vi "Write S6F1.vi"(8 "error in (no error)":errorcluster, 10 "S6F1":T1, 11 "33-Update Trace Data in":refnum<class "33-Update Trace Data.lvclass">) -> (0 "error out":errorcluster, 3 "33-Update Trace Data out":refnum<class "33-Update Trace Data.lvclass">)   [LabVIEW 2020, in "SECS Scenarios.lvlib" / "33-Update Trace Data.lvclass"]
uses:
  33-Update Trace Data.lvclass
  SECS Communication/S6 Message Class/S6F1.ctl
  SECS Communication/SECS-II Class/Format Code.ctl
  33-Update Trace Data.lvclass/33-Update Trace Data.ctl
  SECS Communication/SECS-II Class/SECS-II Class.lvclass
  SECS Communication/S6 Message Class/S6 Message Class.lvclass
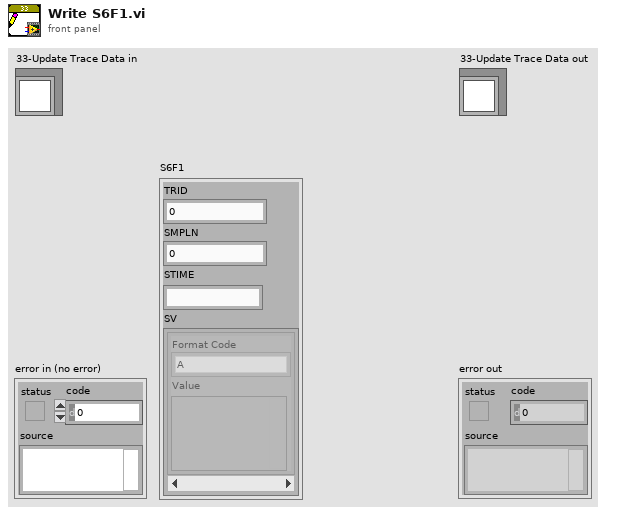
[diagram p1: front panel]
types:
  T1 = typedef "SECS Communication.lvlib/S6 Message Class.lvclass/S6F1.ctl" = cluster{"TRID":u32, "SMPLN":u32, "STIME":string, "SV":cluster{"Format Code":T2, "Value":variant}[]}
  T2 = typedef "SECS Communication.lvlib/SECS-II Class.lvclass/Format Code.ctl" = enum16{"L", "A", "B", "Boolean", "J", "I1", "I2", "I4", "I8", "U1", "U2", "U4", "U8", "F4", "F8", "Char"}
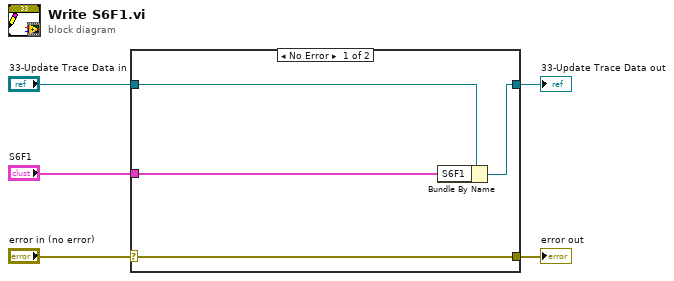
[diagram p0: block diagram]
diagram:
  n1 = case shown="No Error" "error in (no error)" {
    selector: "error in (no error)" -> [w9 w10]
    tunnel: [w9 w10] -> w4
    tunnel: [w7 w11] -> w2
    tunnel: "33-Update Trace Data in" -> [w8 w11]
    tunnel: "S6F1" -> [w6 _]
    frame No Error {
      n2 = Bundle By Name(cluster=w8, "S6F1"=w6) -> (w7:refnum<class "33-Update Trace Data.lvclass">)
    }
    frame Error {
    }
  }
  "error out" <- w4
  "33-Update Trace Data out" <- w2
